vi "plot_update.vi"(0 "data":sgl[](array[numeric]) format="%.2f", 1 "data length":i32, 2 "x zoom factor":dbl format="%.2f", 3 "X range min":sgl format="%.2f", 4 "X range max":sgl format="%.2f", 5 "error in (no error)":errorcluster, 6 "graph ref":T1, 7 "X Scale.Name Label.Text":string, 8 "y min value":sgl format="%.2f", 9 "Y Scale.Name Label.Text":string, 10 "y max value":sgl format="%.2f", 11 "error rangeViolation":bool=TRUE, 12 "autoScale Y":bool, 13 "data idxStart":i32) -> (14 "dataVal max":sgl format="%.2f", 15 "dataVal min":sgl format="%.2f", 19 "error out":errorcluster)   [LabVIEW 2010, in "OSA.lvclass"]
doc: "Reads the contents of a <B>Thorlabs_OSA_64</B> object.\n\n[GOOP 1.0]"
uses:
  OSA.lvclass
  private/graph_intensity.ctl
panel:
  out "double precision float":dbl format="%^.4e"
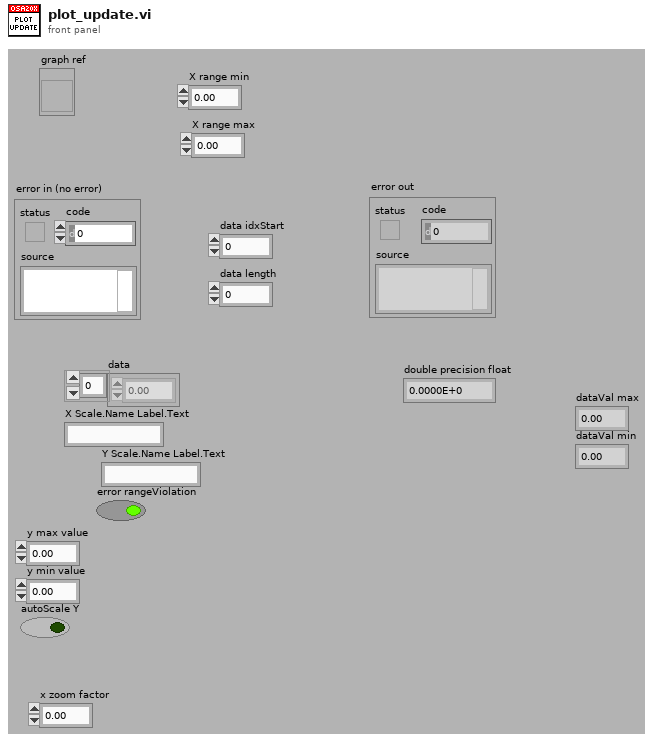
[diagram p1: front panel]
types:
  T1 = typedef "OSA.lvclass/graph_intensity.ctl" = refnum<vi>
  T2 = typedef "LVBoundsTypeDef.ctl" = cluster{"Width":u32, "Height":u32}
  T3 = cluster{"Name":string, "Color":u32, "Hair Style":u8, "Point Style":u8, "Name Visible":bool, "Trackable":bool, "Lock Style":u32, "Plot Number":u32, "Marker Index":i32, "Location":cluster{"X":dbl, "Y":dbl}}[]
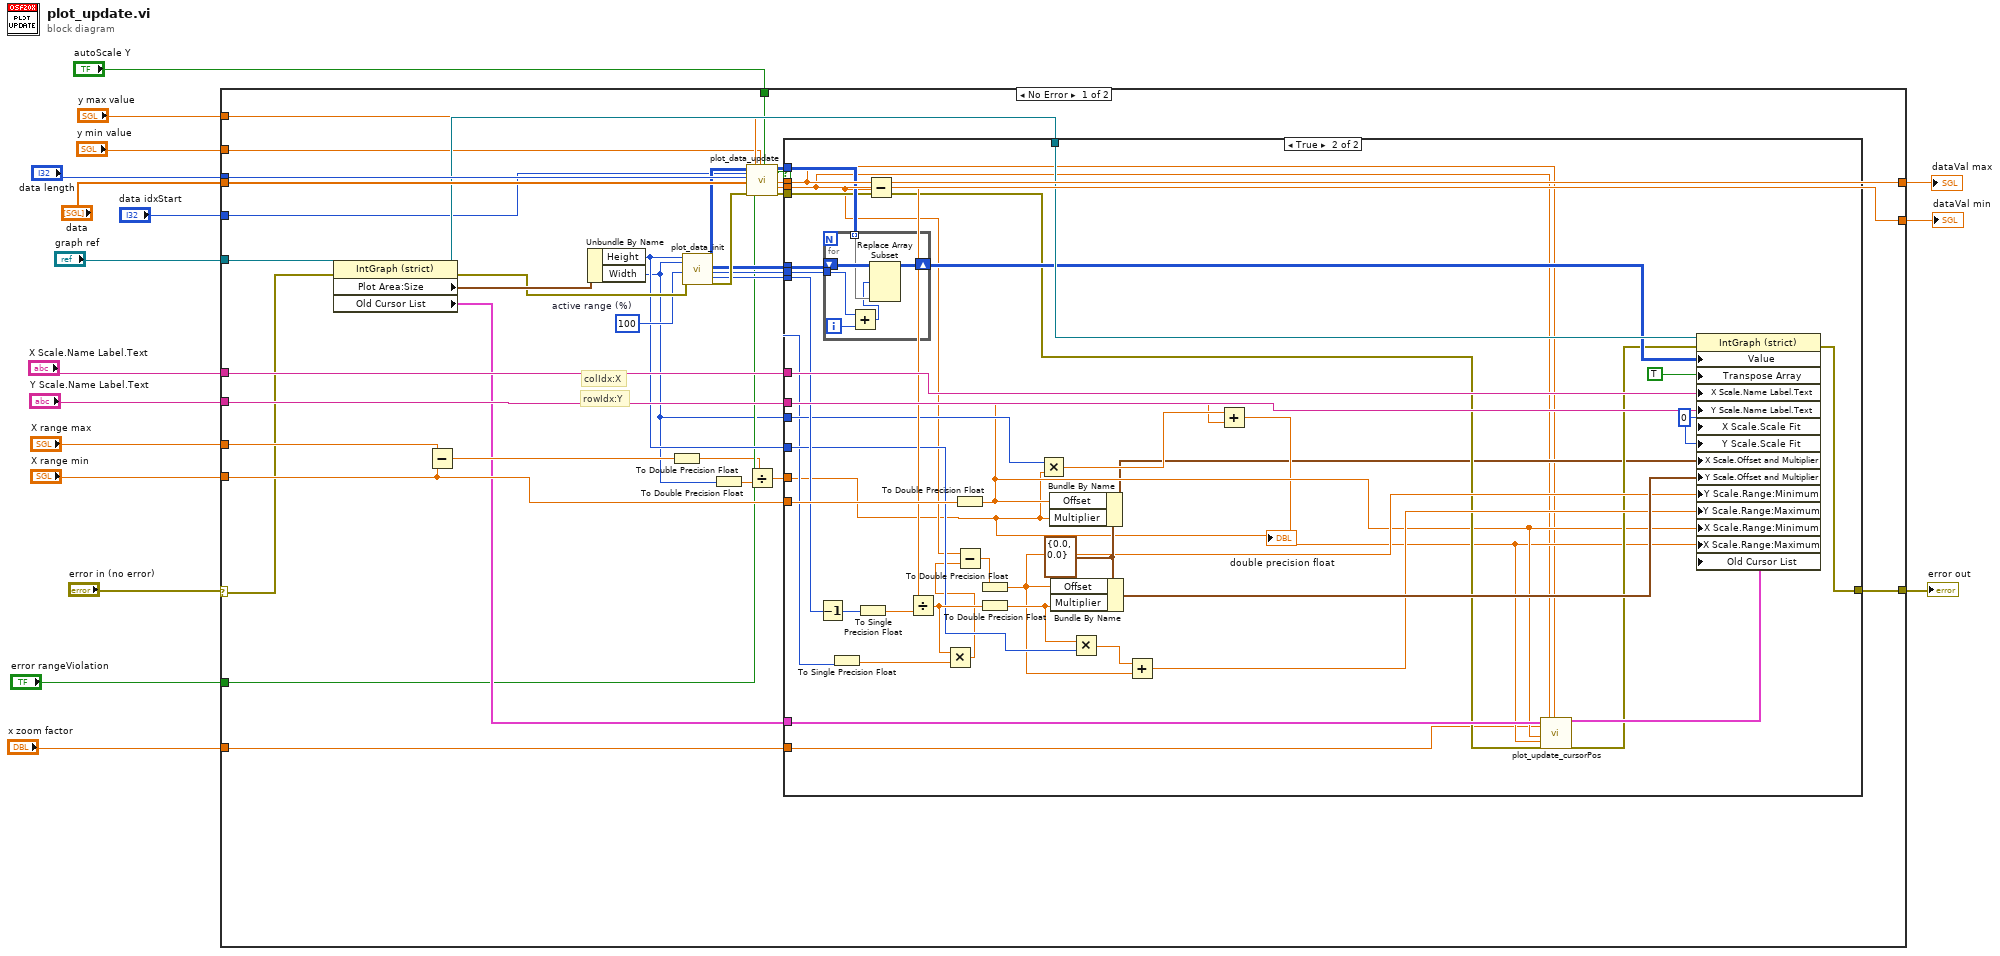
[diagram p0: block diagram]
diagram:
  n1 = case shown="No Error" "error in (no error)" {
    selector: "error in (no error)" -> [w35 w102]
    tunnel: [w46 w102] -> w17
    tunnel: "graph ref" -> [w20 _]
    tunnel: "data length" -> [w50 _]
    tunnel: "data" -> [w49 _]
    tunnel: "X Scale.Name Label.Text" -> [w43 _]
    tunnel: "Y Scale.Name Label.Text" -> [w42 _]
    tunnel: "X range min" -> [w40 _]
    tunnel: "X range max" -> [w41 _]
    tunnel: "error rangeViolation" -> [w28 _]
    tunnel: "y max value" -> [w26 w101]
    tunnel: "y min value" -> [w25 w100]
    tunnel: "autoScale Y" -> [w24 _]
    tunnel: [w36 w101] -> w4
    tunnel: [w23 w100] -> w3
    tunnel: "x zoom factor" -> [w22 _]
    tunnel: "data idxStart" -> [w21 _]
    frame No Error {
      w48 = u32 100  # active range (%)
      # "colIdx:X"
      # "rowIdx:Y"
      # "Put your own code here"
      n2 = property class="IntGraph (strict)"(reference=w20, error in=w35) -> (reference out=w47:T1, error out=w52:errorcluster, "Plot Area:Size"=w53:T2, "Old Cursor List"=w30:T3)
      n3 = Subtract(x=w41, y=w40) -> (x-y=w39:sgl)
      n4 = Unbundle By Name(w53) -> ("Height"=w32:u32, "Width"=w19:u32)
      n5 = To Double Precision Float(number=w39) -> (double precision float=w18:dbl)
      n6 = call "plot_data_init.vi"("pixels Y"=w32, "pixels X"=w19, "active range (%)"=w48, "error in (no error)"=w52) -> ("plot data active"=w33:i32[][], "plot data"=w44:i32[][], "Y active idx start"=w31:i32, "Y active length"=w34:i32, "error out"=w51:errorcluster)  [unwired: 11 in]
      n7 = To Double Precision Float(number=w19) -> (double precision float=w38:dbl)
      n8 = call "plot_data_update.vi"("plotData"=w33, "idx start"=w21, "length"=w50, "AcqData"=w49, "error in (no error)"=w51, "max value"=w26, "error rangeViolation"=w28, "min value"=w25, "autoScale Y"=w24) -> ("plotData out"=w45:i32[][], "updated"=w27:bool, "dataVal max"=w36:sgl, "dataVal min"=w23:sgl, "error out"=w29:errorcluster)  [unwired: 3 in, 3 out]
      n9 = Divide(x=w18, y=w38) -> (x/y=w37:dbl)
      n10 = case shown="True" w27 {
        tunnel: w47 -> [_ w93]
        tunnel: [w54 w92] -> w46
        tunnel: w45 -> [_ w91]
        tunnel: w44 -> [_ w90]
        tunnel: w43 -> [_ w89]
        tunnel: w42 -> [_ w88]
        tunnel: w40 -> [_ w87]
        tunnel: w37 -> [_ w55]
        tunnel: w36 -> [_ w58]
        tunnel: w34 -> [_ w83]
        tunnel: w19 -> [_ w78]
        tunnel: w32 -> [_ w77]
        tunnel: w31 -> [_ w73]
        tunnel: w23 -> [_ w57]
        tunnel: w30 -> [_ w66]
        tunnel: w29 -> [w54 w64]
        tunnel: w22 -> [_ w56]
        frame False {
        }
        frame True {
          w59 = u8 0 ("X Scale.Scale Fit")
          w86 = cluster{"Offset":dbl, "Multiplier":dbl} {"Offset"=0.0, "Multiplier"=0.0} ("X Scale.Offset and Multiplier")
          n11 = Decrement(x=w83) -> (x-1=w70:i32)
          n12 = for {
            tunnel: w91 -> [w98] mode=indexing
            shift-right: [w97] -> w79
            shift-left: w90 -> [w99]
            tunnel: w73 -> [w95]
            i -> [w96]
            n13 = Add(x=w95, y=w96) -> (x+y=w94:i32)
            n14 = Replace Array Subset(array=w99, new element=w98, index (row)=w94) -> (w97:i32[][])  [unwired: 1 in]
          }
          n15 = To Single Precision Float(number=w73) -> (single precision float=w82:sgl)
          n16 = To Single Precision Float(number=w70) -> (single precision float=w81:sgl)
          n17 = Subtract(x=w58, y=w57) -> (x-y=w84:sgl)
          n18 = Divide(x=w84, y=w81) -> (x/y=w80:sgl)
          n19 = Multiply(x=w80, y=w82) -> (x*y=w72:sgl)
          n20 = To Double Precision Float(number=w87) -> (double precision float=w62:dbl)
          n21 = Subtract(x=w57, y=w72) -> (x-y=w71:sgl)
          n22 = To Double Precision Float(number=w71) -> (double precision float=w69:dbl)
          n23 = To Double Precision Float(number=w80) -> (double precision float=w74:dbl)
          n24 = Multiply(x=w78, y=w55) -> (x*y=w75:dbl)
          n25 = Bundle By Name(cluster=w86, "Offset"=w62, "Multiplier"=w55) -> (w60:cluster{"Offset":dbl, "Multiplier":dbl})
          n26 = Bundle By Name(cluster=w86, "Offset"=w69, "Multiplier"=w74) -> (w85:cluster{"Offset":dbl, "Multiplier":dbl})
          n27 = Multiply(x=w74, y=w77) -> (x*y=w76:dbl)
          n28 = Add(x=w76, y=w69) -> (x+y=w68:dbl)
          n29 = Add(x=w75, y=w62) -> (x+y=w61:dbl)
          n30 = call "plot_update_cursorPos.vi"("cursor list"=w66, "x zoom factor"=w56, "x min"=w62, "x max"=w61, "error in (no error)"=w64, "y max"=w57, "y min"=w58) -> ("cursor list out"=w65:T3, "error out"=w63:errorcluster)  [unwired: 11 in]
          n31 = property class="IntGraph (strict)"(reference=w93, error in=w63, "Value"=w79, "Transpose Array"=TRUE, "X Scale.Name Label.Text"=w89, "Y Scale.Name Label.Text"=w88, "X Scale.Scale Fit"=w59, "Y Scale.Scale Fit"=w59, "X Scale.Offset and Multiplier"=w60, "Y Scale.Offset and Multiplier"=w85, "Y Scale.Range:Minimum"=w69, "Y Scale.Range:Maximum"=w68, "X Scale.Range:Minimum"=w62, "X Scale.Range:Maximum"=w61, "Old Cursor List"=w65) -> (error out=w92:errorcluster)  [unwired: 1 out]
          "double precision float" <- w55
        }
      }
    }
    frame Error {
      # "Error"
    }
  }
  "error out" <- w17
  "dataVal max" <- w4
  "dataVal min" <- w3
